vi "HMI --Run Command on HMI.vi"(4 "Baud":u32=9600, 5 "Enable?(Default:T)":bool=TRUE, 6 "timeOut(ms)":u32=5000, 7 "Dialog In":refnum<vi>, 8 "error in (no error)":errorcluster, 9 "expectMsg":string="UUCÞ°Ø", 10 "Command":string="UUC!ð˜", 11 "VISA resource name":refnum<visa-resource-name>="COM7") -> (0 "error out":errorcluster, 2 "detected?":bool, 3 "Read out":string)   [LabVIEW 2011]
uses:
  <vilib>/Instr/_visa.llb/VISA Configure Serial Port (Instr).vi
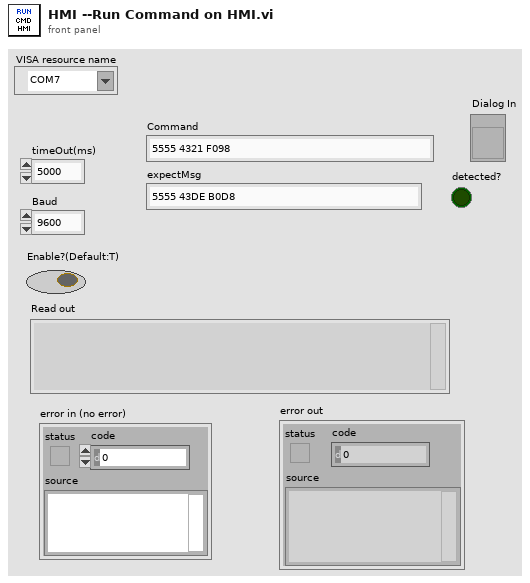
[diagram p1: front panel]
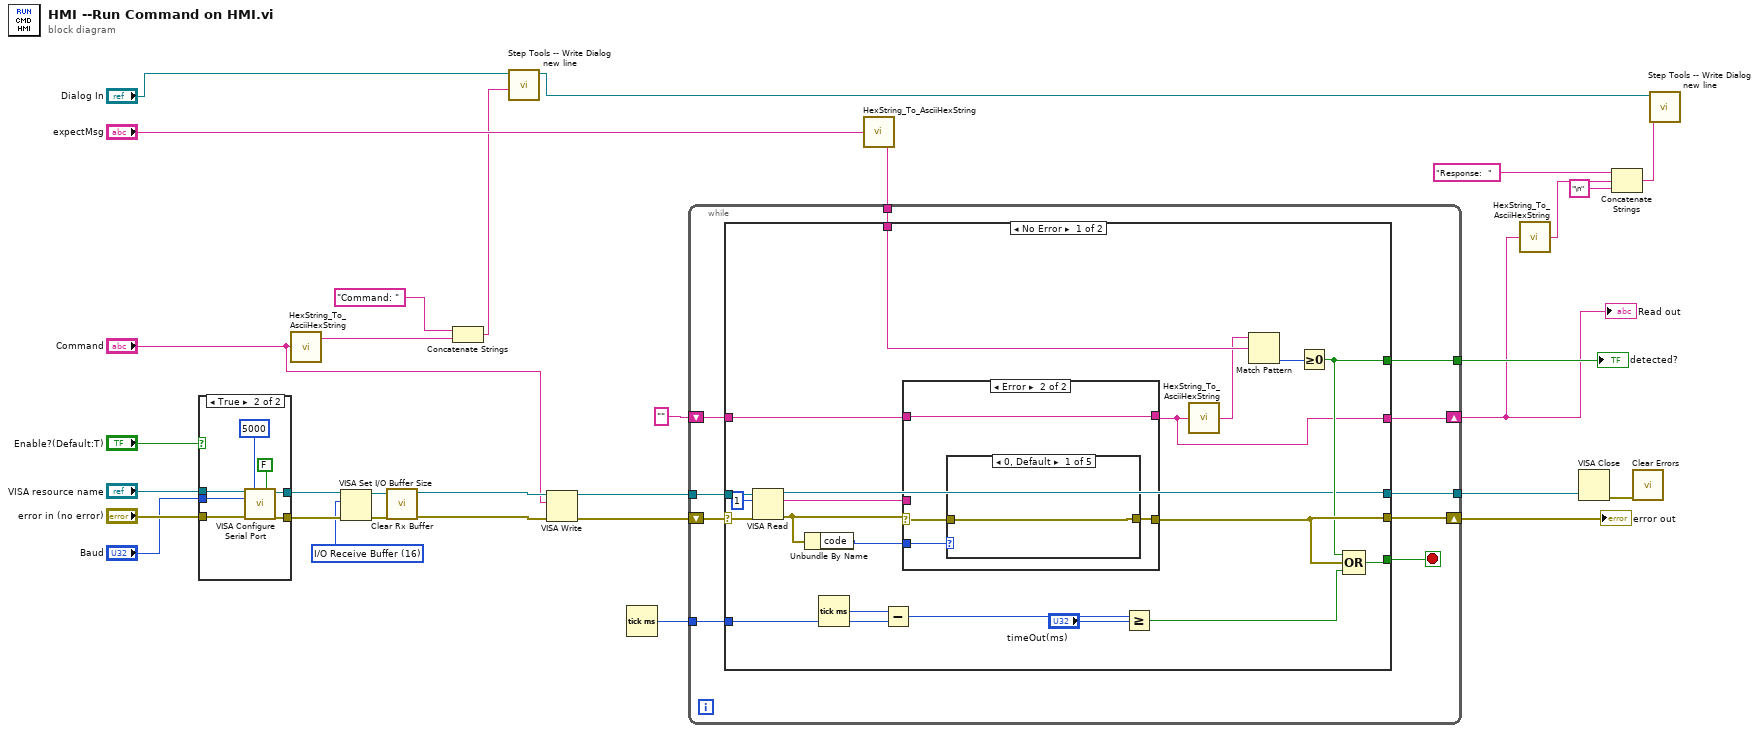
[diagram p0: block diagram]
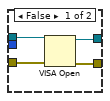
[diagram p2: hidden frame]
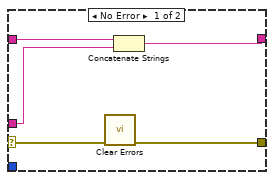
[diagram p3: hidden frame]
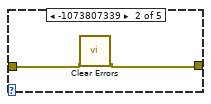
[diagram p4: hidden frame]
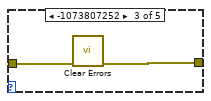
[diagram p5: hidden frame]
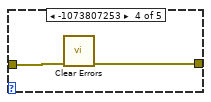
[diagram p6: hidden frame]
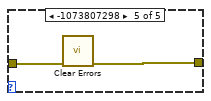
[diagram p7: hidden frame]
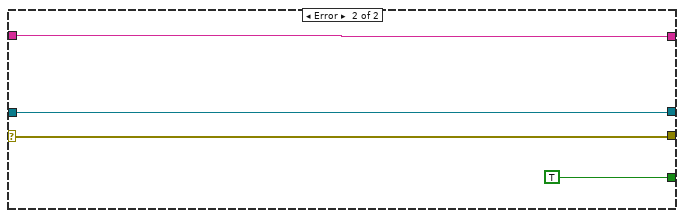
[diagram p8: hidden frame]
diagram:
  w1 = u16 16 items=["I/O Receive Buffer"=16, "I/O Transmit Buffer"=32, "I/O Receive and Transmit Buffer"=48] ("Mask")
  n1 = case shown="True" "Enable?(Default:T)" {
    tunnel: "error in (no error)" -> [w33 w43]
    tunnel: "VISA resource name" -> [w34 w42]
    tunnel: "Baud" -> [_ w39]
    tunnel: [w36 w38] -> w25
    tunnel: [w35 w37] -> w24
    frame False {
      n2 = VISA Open(error in (no error)=w33, VISA resource name=w34) -> (VISA resource name=w35:refnum<visa-resource-name>, error out=w36:errorcluster)  [unwired: 3 in]
    }
    frame True {
      n3 = call-poly "VISA Configure Serial Port"("VISA resource name"=w42, "timeout (10sec)"=u32 5000, "Enable Termination\nChar (T)"=FALSE ("Enable Termination\nChar (T)"), "baud rate (9600)"=w39, "error in (no error)"=w43) -> ("VISA resource name out"=w37:refnum<visa-resource-name>, "error out"=w38:errorcluster)  [unwired: 9 in]
    }
  }
  n4 = call "HexString_To_AsciiHexString.vi"("HexString"="Command") -> ("AsciiHexString"=w18:string)
  n5 = VISA Set I/O Buffer Size(VISA resource name=w24, mask (16)=w1, error in (no error)=w25) -> (VISA resource name out=w3:refnum<visa-resource-name>, error out=w2:errorcluster)  [unwired: 1 in]
  n6 = call "Clear Rx Buffer.vi"("error in"=w2, "Com Port"=w3) -> ("error out"=w10:errorcluster, "Com Port out"=w9:refnum<visa-resource-name>)  [unwired: 8 out]
  n7 = Concatenate Strings("Command: " ("string"), w18) -> (w7:string)
  n8 = call "Step Tools -- Write Dialog new line.vi"("String For Write"=w7, "Dialog In"="Dialog In") -> ("Dialog Out"=w5:refnum<vi>)  [unwired: 6 in, 1 out]
  n9 = VISA Write(VISA resource name=w9, write buffer="Command", error in (no error)=w10) -> (VISA resource name out=w30:refnum<visa-resource-name>, error out=w19:errorcluster)  [unwired: 1 out]
  n10 = Tick Count (ms)() -> (millisecond timer value=w28:u32)
  n11 = call "HexString_To_AsciiHexString.vi"("HexString"="expectMsg") -> ("AsciiHexString"=w13:string)
  n12 = while {
    tunnel: w30 -> [w53]
    tunnel: [w52] -> w29
    shift-right: [w48] -> w12
    shift-left: "" -> [w49]
    tunnel: w28 -> [w47]
    tunnel: [w46] -> w26
    tunnel: w13 -> [w45]
    shift-right: [w44] -> w4
    shift-left: w19 -> [w51]
    stop <- w50 stop-if-true
    n13 = case shown="No Error" w51 {
      selector: w51 -> [w61 w94]
      tunnel: [w66 w94] -> w44
      tunnel: w53 -> [w63 w95]
      tunnel: [w64 w95] -> w52
      tunnel: [w67 TRUE] -> w50
      tunnel: w49 -> [w59 w92]
      tunnel: [w56 w92] -> w48
      tunnel: w47 -> [w71 _]
      tunnel: [w65 _] -> w46
      tunnel: w45 -> [w57 _]
      frame No Error {
        n14 = VISA Read(VISA resource name=w63, byte count=u32 1, error in (no error)=w61) -> (VISA resource name out=w64:refnum<visa-resource-name>, read buffer=w54:string, error out=w60:errorcluster)  [unwired: 1 out]
        n15 = Unbundle By Name(w60) -> ("code"=w58:i32)
        n16 = Tick Count (ms)() -> (millisecond timer value=w72:u32)
        n17 = Subtract(x=w72, y=w71) -> (x-y=w70:u32)
        n18 = case shown="Error" w60 {
          selector: w60 -> [w75 w82]
          tunnel: [w74 w81] -> w66
          tunnel: w54 -> [w78 _]
          tunnel: w59 -> [w77 w79]
          tunnel: [w76 w79] -> w56
          tunnel: w58 -> [_ w80]
          frame No Error {
            n19 = call <vilib>:"Clear Errors.vi"("error in (no error)"=w75) -> ("error out"=w74:errorcluster)  [unwired: 6 in]
            n20 = Concatenate Strings(w77, w78) -> (w76:string)
          }
          frame Error {
            n21 = case shown="0, Default" w80 {
              tunnel: w82 -> [w83 w85 w87 w89 w91]
              tunnel: [w83 w84 w86 w88 w90] -> w81
              frame 0, Default {
              }
              frame -1073807339 {
                n22 = call <vilib>:"Clear Errors.vi"("error in (no error)"=w85) -> ("error out"=w84:errorcluster)  [unwired: 6 in]
              }
              frame -1073807252 {
                n23 = call <vilib>:"Clear Errors.vi"("error in (no error)"=w87) -> ("error out"=w86:errorcluster)  [unwired: 6 in]
              }
              frame -1073807253 {
                n24 = call <vilib>:"Clear Errors.vi"("error in (no error)"=w89) -> ("error out"=w88:errorcluster)  [unwired: 6 in]
              }
              frame -1073807298 {
                n25 = call <vilib>:"Clear Errors.vi"("error in (no error)"=w91) -> ("error out"=w90:errorcluster)  [unwired: 6 in]
              }
            }
          }
        }
        n26 = Greater Or Equal?(x=w70, y="timeOut(ms)") -> (x >= y?=w68:bool)
        n27 = call "HexString_To_AsciiHexString.vi"("HexString"=w56) -> ("AsciiHexString"=w55:string)
        n28 = Match Pattern(string=w55, regular expression=w57) -> (offset past match=w73:i32)  [unwired: 1 in, 3 out]
        n29 = Greater Or Equal To 0?(x=w73) -> (x >= 0?=w65:bool)
        n30 = Compound Arithmetic op=OR(w65, w66, w68) -> (w67:bool)
      }
      frame Error {
      }
    }
  }
  "error out" <- w4
  "Read out" <- w12
  "detected?" <- w26
  n31 = call "HexString_To_AsciiHexString.vi"("HexString"=w12) -> ("AsciiHexString"=w11:string)
  n32 = VISA Close(VISA resource name=w29) -> (error out=w16:errorcluster)  [unwired: 1 in]
  n33 = Concatenate Strings("Response:  " ("string"), w11, "\n" ("string")) -> (w22:string)
  n34 = call <vilib>:"Clear Errors.vi"("error in (no error)"=w16) -> ()  [unwired: 6 in, 1 out]
  n35 = call "Step Tools -- Write Dialog new line.vi"("String For Write"=w22, "Dialog In"=w5) -> ()  [unwired: 6 in, 2 out]
